vi "Deviation Signal Chart.vi"() -> ()   [LabVIEW 2013]
panel:
  out "Deviation Chart":dbl(graph)
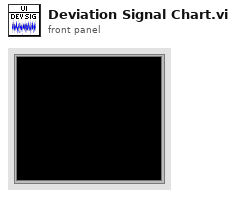
[diagram p1: front panel]
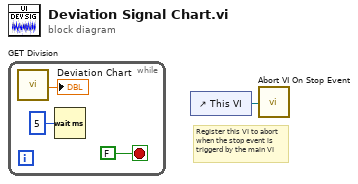
[diagram p0: block diagram]
diagram:
  # "Register this VI to abort\nwhen the stop event is\ntriggerd by the main VI"
  n1 = while {
    stop <- FALSE stop-if-true
    n2 = call "GET Division.vi"() -> ("Division"=→"Deviation Chart":dbl)
    n3 = Wait (ms)(milliseconds to wait=u32 5) -> ()  [unwired: 1 out]
  }
  n4 = control-ref of="This VI"() -> (w1:refnum<vi>)
  n5 = call "Abort VI On Stop Event.vi"("VI Reference"=w1) -> ()
